vi "Main v0.1.vi"() -> ()   [LabVIEW 2017]
doc: "This template is for the Queued Message Handler design pattern.\n\nThe Event Handling Loop generates messages based on user interface actions.\n\nThe Message Handling Loop processes messages generated by the Event Handling Loop, or by other messages. The messages are string values, so new messages can be added easily to the Message Cases case structure in the Message Handling Loop. Each message cluster can also provide an optional value for Message Data, which is a variant that can be converted to whatever message-specific data is required."
uses:
  Controls/Main Tabs.ctl
  Controls/Auto.ctl
  Controls/UI Data.ctl
  support/Message Queue/Enqueue Message (Single).vi
  <vilib>/Utility/error.llb/Error Cluster From Error Code.vi
  <vilib>/ErrorRing/Error Ring.xnode
  support/Message Queue/Message Queue.lvlib
  support/User Event - Stop/User Event - Stop.lvlib
panel:
  out "Date-Time":string caption="Dip-Tube Assembly Automation (HMI) v0.1"
  out "Main Tab":T1
  in  "Autocycle":T2
  in  "Manual":bool
  in  "Parameters":bool
  in  "Maintenance":bool
  in  "Save Para":bool
  in  "Home Para":bool
  in  "ParaTab":T3(tab)
  in  "StopperRearDelay":dbl format="%#.2f"
  in  "StopperFrontDelay":dbl format="%#.2f"
  in  "MaxAlarms":dbl caption="Max Alarms in 1 Minute" format="%#.2f"
  in  "MaxConsecutive":dbl caption="Max Consecutive Alarms" format="%#.2f"
  in  "Gate Close Delay":dbl format="%#.2f"
  in  "Gate Open Delay":dbl format="%#.2f"
  in  "BF Off Delay":dbl format="%#.2f"
  in  "BF On Delay":dbl format="%#.2f"
  in  "DelayAfterReject":dbl format="%#.2f"
  in  "MeasurementTime":dbl format="%#.2f"
  in  "DelayAfterMesFront":dbl format="%#.2f"
  in  "DelayAfterCut":dbl format="%#.2f"
  in  "DelayAfterCutClamp":dbl format="%#.2f"
  in  "DelayAfterInsClamp":dbl format="%#.2f"
  in  "DelayToClose":dbl format="%#.2f"
  in  "DelayToOpen":dbl format="%#.2f"
  in  "DelayAfterInsertion":dbl format="%#.2f"
  in  "DelayBeforeInsertion":dbl format="%#.2f"
  in  "AgitatorUpTime":dbl format="%#.2f"
  in  "AgitatorDownTime":dbl format="%#.2f"
  in  "All IO":bool
  in  "Stats":bool
  in  "Home AC":bool
  out "Status":string
  out "Count":dbl format="%06.0f"
  out "Count 3":dbl caption="Cycle Time" format="%0.2f"
  out "Count 2":dbl caption="Rejects" format="%06.0f"
  in  "Statuses":string[][](table)
  in  "Exit":bool
  # "Vision Harmony Dip-Tube Assembly Automation"
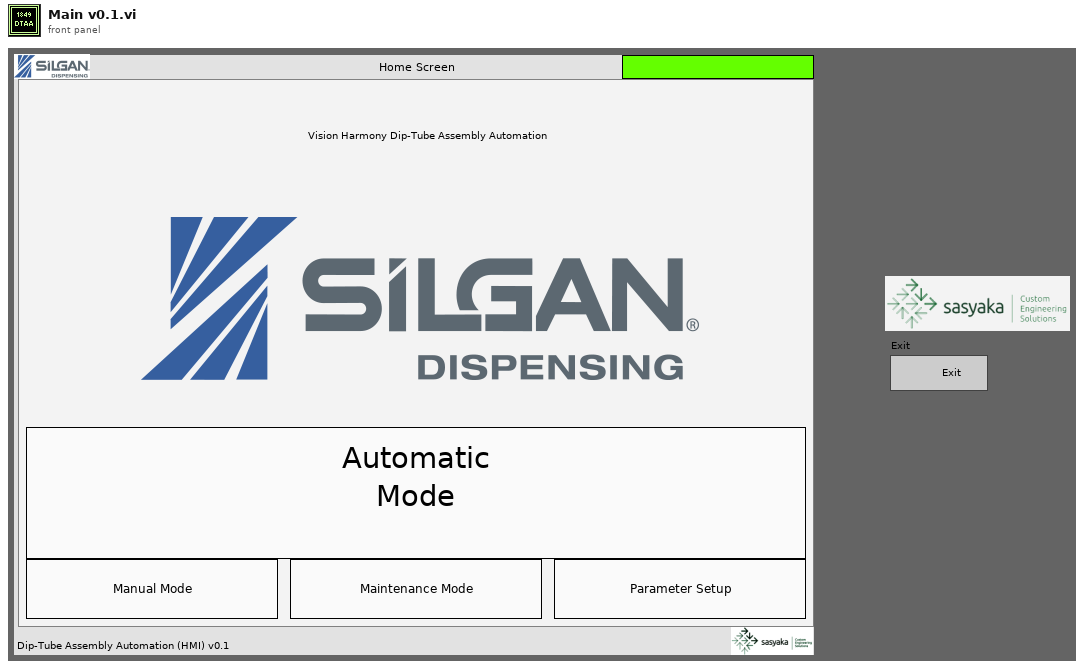
[diagram p1: front panel]
types:
  T1 = typedef "Main Tabs.ctl" = enum32{"Home Screen", "Parameter Setup", "Manual Mode", "Autocycle"}
  T2 = typedef "Auto.ctl" = bool
  T3 = enum32{"General & Indexing", "Bowl Feeder & Pump Conveyor", "Cutting, Measurement & Rejection", "Tube Feeder & Insertion"}
  T4 = typedef "UI Data.ctl" = cluster{"Main Tab":refnum<vi>}
  T5 = typedef "Message Queue.lvlib/All Message Queues.ctl" = cluster{"UI":refnum<queue>}
  T6 = enum8{"Enabled", "Disabled", "Disabled and Grayed Out"}
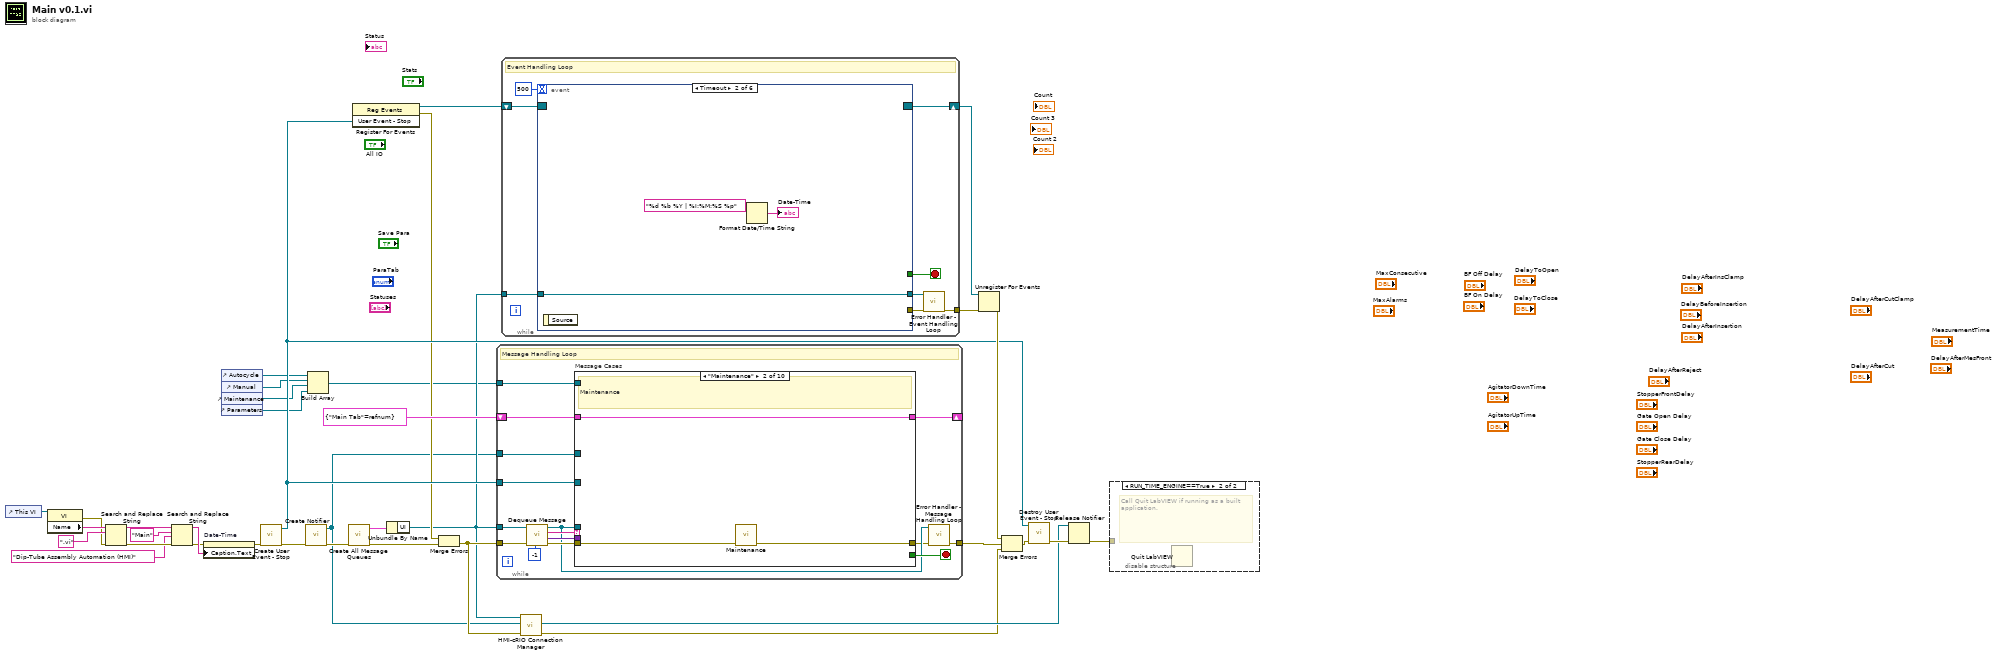
[diagram p0: block diagram]
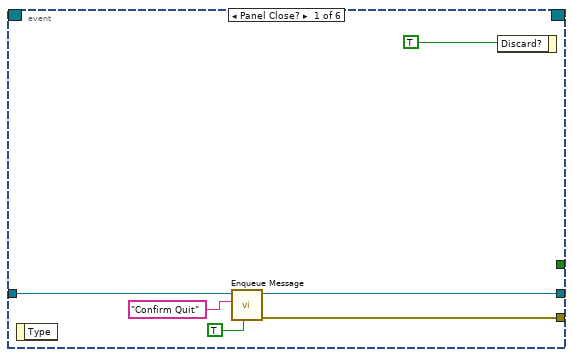
[diagram p2: hidden frame]
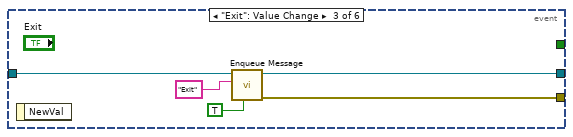
[diagram p3: hidden frame]
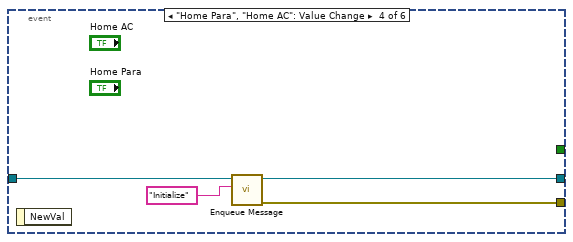
[diagram p4: hidden frame]
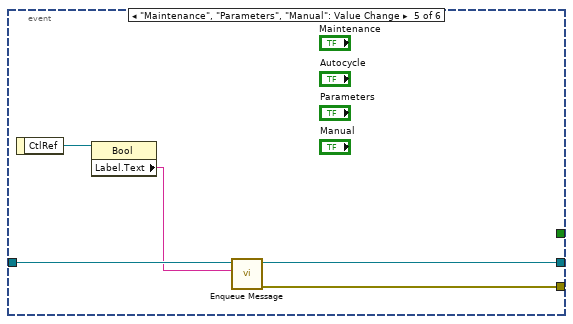
[diagram p5: hidden frame]
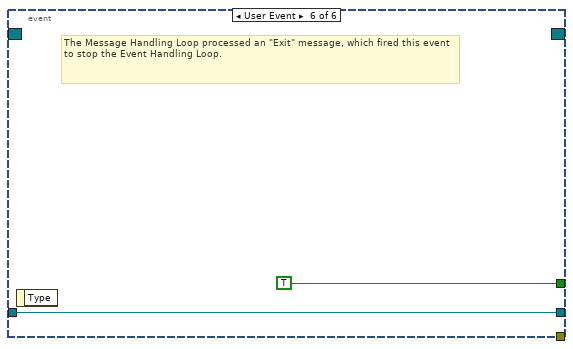
[diagram p6: hidden frame]
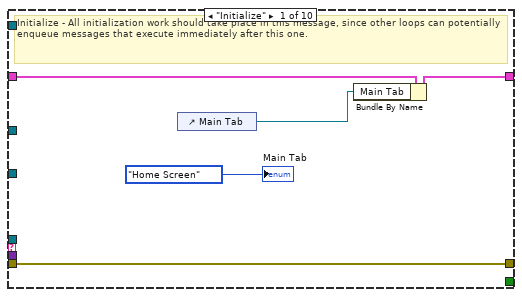
[diagram p7: hidden frame]
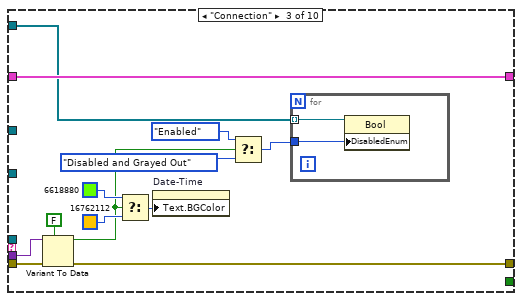
[diagram p8: hidden frame]
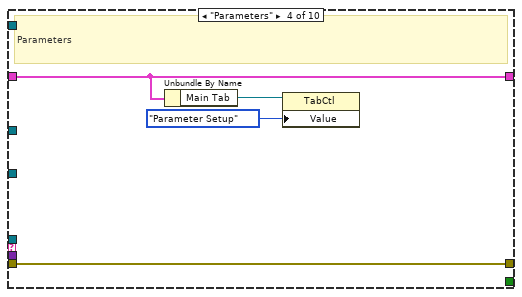
[diagram p9: hidden frame]
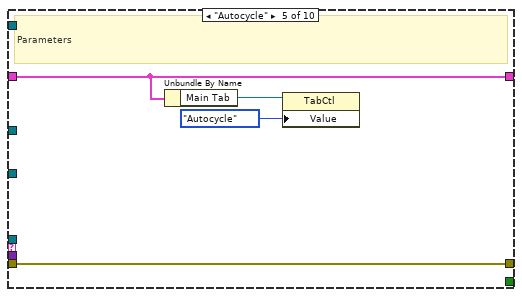
[diagram p10: hidden frame]
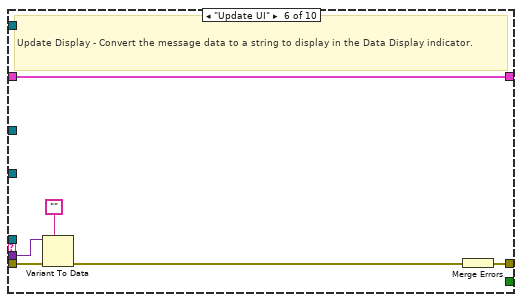
[diagram p11: hidden frame]
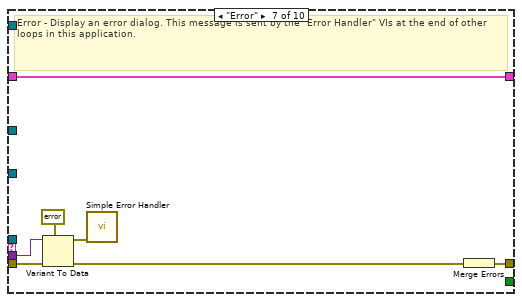
[diagram p12: hidden frame]
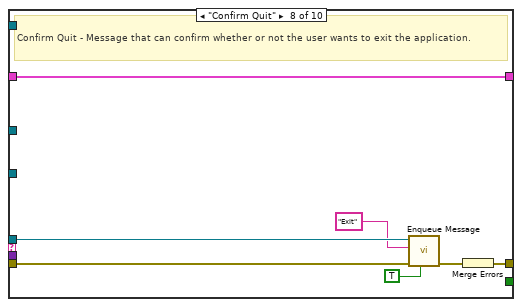
[diagram p13: hidden frame]
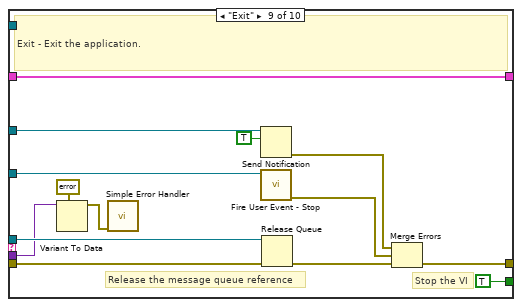
[diagram p14: hidden frame]
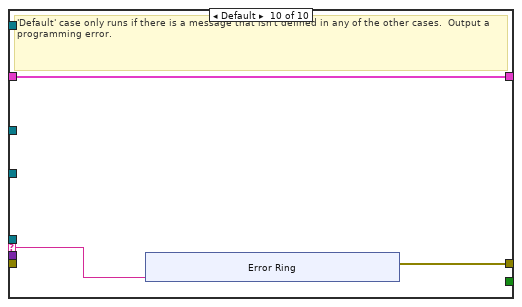
[diagram p15: hidden frame]
diagram:
  n1 = control-ref of="This VI"() -> (w5:refnum<vi>)
  n2 = property class="VI"(reference=w5) -> (error out=w4:errorcluster, "Name"=w11:string)  [unwired: 1 in, 1 out]
  n3 = Search and Replace String(input string=w11, search string=".vi", error in=w4) -> (result string=w9:string, error out=w8:errorcluster)  [unwired: 5 in, 2 out]
  n4 = Search and Replace String(input string=w9, search string="Main", replace string="Dip-Tube Assembly Automation (HMI)" ("replace string (\"\")"), error in=w8) -> (result string=w3:string, error out=w2:errorcluster)  [unwired: 4 in, 2 out]
  n5 = property on="Date-Time" class="Str"(error in=w2, "Caption.Text"=w3) -> (error out=w1:errorcluster)  [unwired: 1 in, 1 out]
  n6 = control-ref of="Autocycle"() -> (w16:refnum<vi>)
  n7 = control-ref of="Manual"() -> (w15:refnum<vi>)
  n8 = control-ref of="Maintenance"() -> (w14:refnum<vi>)
  n9 = control-ref of="Parameters"() -> (w13:refnum<vi>)
  n10 = call "Create User Event - Stop.vi"("error in (no error)"=w1) -> ("error out"=w23:errorcluster, "User Event - Stop"=w27:refnum<user-event>)  [unwired: 9 in]
  n11 = call "Create Notifier.vi"("error in (no error)"=w23) -> ("error out"=w22:errorcluster, "notifier out"=w17:refnum<notifier>)  [unwired: 9 in]
  n12 = Build Array(w16, w15, w14, w13) -> (w12:refnum<vi>[])
  n13 = call "Create All Message Queues.vi"("error in (no error)"=w22) -> ("error out"=w36:errorcluster, "Message Queues out"=w35:T5)  [unwired: 9 in]
  n14 = register-events(w27) -> (reference out=w28:refnum<event-registration>, error out=w26:errorcluster)  [unwired: 2 in]
  n15 = Unbundle By Name(w35) -> ("UI"=w24:refnum<queue>)
  n16 = Merge Errors(w26, w36) -> (w25:errorcluster)
  n17 = while {
    tunnel: w24 -> [w43]
    shift-right: [w50] -> _
    shift-left: T4 {"Main Tab"=refnum} ("Data Cluster") -> [w51]
    tunnel: w27 -> [w48]
    tunnel: w25 -> [w47]
    tunnel: [w41] -> w34
    tunnel: w17 -> [w38]
    tunnel: w12 -> [w37]
    stop <- w49 stop-if-true
    # "Message Handling Loop"
    n18 = call "Dequeue Message.vi"("timeout"=-1, "error in (no error)"=w47, "Message Queue"=w43) -> ("error out"=w46:errorcluster, "Message Data"=w44:variant, "Message"=w45:string, "dup Message Queue"=w42:refnum<queue>)  [unwired: 5 in]
    n19 = case "Message Cases" shown="\"Maintenance\"" w45 {
      selector: w45 -> [_ _ _ _ _ _ _ _ _ w117]
      tunnel: w42 -> [_ _ _ _ _ _ _ w98 w116 _]
      tunnel: w46 -> [w56 w58 w70 w78 w82 w86 w95 w102 w109 _]
      tunnel: [w56 w57 w69 w78 w82 w87 w89 w100 w112 w118] -> w40
      tunnel: w51 -> [w55 w59 w72 w77 w81 w88 w94 w101 w115 w119]
      tunnel: [w54 w59 w72 w77 w81 w88 w94 w101 w115 w119] -> w50
      tunnel: [_ _ _ _ _ _ _ _ TRUE _] -> w49
      tunnel: w44 -> [_ _ w68 _ _ w85 w93 _ w106 _]
      tunnel: w48 -> [_ _ _ _ _ _ _ _ w111 _]
      tunnel: w38 -> [_ _ _ _ _ _ _ _ w105 _]
      tunnel: w37 -> [_ _ w64 _ _ _ _ _ _ _]
      frame "Initialize" {
        # "Initialize - All initialization work should take place in this message, since other loops can potentially enqueue messages that execute immediately after this one."
        n20 = control-ref of="Main Tab"() -> (w53:refnum<vi>)
        n21 = Bundle By Name(cluster=w55, "Main Tab"=w53) -> (w54:T4)
        "Main Tab" <- Main_Tabs."Home Screen" ("Main Tab")
      }
      frame "Maintenance" {
        # "Maintenance"
        n22 = call "Maintenance.vi"("Error In"=w58) -> ("Error out"=w57:errorcluster)  [unwired: 10 in]
      }
      frame "Connection" {
        n23 = Variant To Data(error in=w70, type=FALSE, Variant=w68) -> (data=w63:bool, error out=w69:errorcluster)
        n24 = Select(t=u32 6618880 ("Text.Text Colors:BG Color"), s=w63, f=u32 16762112 ("Text.Text Colors:BG Color")) -> (s? t:f=w65:u32)
        n25 = property on="Date-Time" class="Str"("Text.BGColor"=w65) -> ()  [unwired: 2 in, 2 out]
        n26 = Select(t=T6."Enabled" ("Disabled"), s=w63, f=T6."Disabled and Grayed Out") -> (s? t:f=w61:T6)
        n27 = for {
          tunnel: w64 -> [w74] mode=indexing
          tunnel: w61 -> [w73]
          n28 = property class="Bool"(reference=w74, "DisabledEnum"=w73) -> ()  [unwired: 1 in, 2 out]
        }
      }
      frame "Parameters" {
        # "Parameters"
        n29 = Unbundle By Name(w77) -> ("Main Tab"=w76:refnum<vi>)
        n30 = property class="TabCtl"(reference=w76, "Value"=Main_Tabs."Parameter Setup" ("Main Tab")) -> ()  [unwired: 1 in, 2 out]
      }
      frame "Autocycle" {
        # "Parameters"
        n31 = Unbundle By Name(w81) -> ("Main Tab"=w80:refnum<vi>)
        n32 = property class="TabCtl"(reference=w80, "Value"=Main_Tabs."Autocycle" ("Main Tab")) -> ()  [unwired: 1 in, 2 out]
      }
      frame "Update UI" {
        # "Update Display - Convert the message data to a string to display in the Data Display indicator."
        n33 = Variant To Data(error in=w86, type="", Variant=w85) -> (error out=w83:errorcluster)  [unwired: 1 out]
        n34 = Merge Errors(w83) -> (w87:errorcluster)
      }
      frame "Error" {
        # "Error - Display an error dialog. This message is sent by the \"Error Handler\" VIs at the end of other loops in this application."
        n35 = Variant To Data(error in=w95, type=errorcluster {"status"=FALSE, "code"=0, "source"=""} ("error constant"), Variant=w93) -> (data=w91:errorcluster, error out=w90:errorcluster)
        n36 = call <vilib>:"Simple Error Handler.vi"("error in (no error)"=w91) -> ()  [unwired: 4 in, 5 out]
        n37 = Merge Errors(w90) -> (w89:errorcluster)
      }
      frame "Confirm Quit" {
        # "Confirm Quit - Message that can confirm whether or not the user wants to exit the application."
        n38 = call-poly "Enqueue Message.vi"("Priority Message? (F)"=TRUE, "error in (no error)"=w102, "Message"="Exit", "Message Queue"=w98) -> ("error out"=w99:errorcluster)  [unwired: 6 in, 1 out]
        n39 = Merge Errors(w99) -> (w100:errorcluster)
      }
      frame "Exit" {
        # "Stop the VI"
        # "Release the message queue reference"
        # "Exit - Exit the application."
        n40 = Variant To Data(type=errorcluster {"status"=FALSE, "code"=0, "source"=""} ("error constant"), Variant=w106) -> (data=w107:errorcluster)  [unwired: 1 in, 1 out]
        n41 = call <vilib>:"Simple Error Handler.vi"("error in (no error)"=w107) -> ()  [unwired: 4 in, 5 out]
        n42 = Send Notification(notification=TRUE, notifier=w105) -> (error out=w103:errorcluster)  [unwired: 1 in, 1 out]
        n43 = call "Fire User Event - Stop.vi"("User Event - Stop"=w111) -> ("error out"=w110:errorcluster)  [unwired: 10 in]
        n44 = Release Queue(queue=w116, error in (no error)=w109) -> (error out=w113:errorcluster)  [unwired: 1 in, 2 out]
        n45 = Merge Errors(w103, w110, w113) -> (w112:errorcluster)
      }
      frame Default {
        # "'Default' case only runs if there is a message that isn't defined in any of the other cases.  Output a programming error."
        n46 = xnode "Error Ring"("parameter 0"=w117) -> ("error out"=w118:errorcluster)
      }
    }
    n47 = call "Error Handler - Message Handling Loop.vi"("error in (no error)"=w40, "Message Queue"=w42) -> ("dup error in"=w41:errorcluster)  [unwired: 8 in, 1 out]
  }
  n48 = while {
    tunnel: w24 -> [w134]
    shift-right: [w132] -> w31
    shift-left: w28 -> [w133]
    tunnel: [w128] -> w29
    stop <- w130 stop-if-true
    # "Event Handling Loop"
    n49 = event shown="[1] Timeout" {
      selector: w133 -> [_ _ _ _ _ _]
      dyn-events: [_ _ _ _ _ _] -> w132
      timeout: 500 -> [_ _ _ _ _ _]
      tunnel: [_ _ _ _ _ TRUE ("Discard?")] -> w130
      tunnel: w134 -> [w139 w143 w148 w152 w157 w159]
      tunnel: [w138 _ w147 w151 w156 _] -> w131
      tunnel: [w137 w143 w146 w150 w155 w159] -> w129
      event Panel Close? {
        n50 = event-data() -> ()  [unwired: 1 in, 1 out]
        n51 = call-poly "Enqueue Message.vi"("Priority Message? (F)"=TRUE, "Message"="Confirm Quit", "Message Queue"=w139) -> ("error out"=w138:errorcluster, "dup Message Queue"=w137:refnum<queue>)  [unwired: 7 in]
        n52 = event-data("Discard?"=TRUE) -> ()  [unwired: 1 in, 1 out]
      }
      event Timeout {
        n53 = event-data() -> ()  [unwired: 1 in, 1 out]
        n54 = Format Date/Time String(time format string (%c)="%d %b %Y | %I:%M:%S %p") -> (date/time string=→"Date-Time":string)  [unwired: 2 in]
      }
      event "Exit": Value Change {
        n55 = event-data() -> ()  [unwired: 1 in, 1 out]
        n56 = call-poly "Enqueue Message.vi"("Priority Message? (F)"=TRUE, "Message"="Exit", "Message Queue"=w148) -> ("error out"=w147:errorcluster, "dup Message Queue"=w146:refnum<queue>)  [unwired: 7 in]
      }
      event "Home Para", "Home AC": Value Change {
        n57 = event-data() -> ()  [unwired: 1 in, 1 out]
        n58 = call-poly "Enqueue Message.vi"("Message"="Initialize", "Message Queue"=w152) -> ("error out"=w151:errorcluster, "dup Message Queue"=w150:refnum<queue>)  [unwired: 8 in]
      }
      event "Maintenance", "Parameters", "Manual": Value Change {
        n59 = event-data() -> ("CtlRef"=w154:refnum<vi>)  [unwired: 1 in]
        n60 = property class="Bool"(reference=w154) -> ("Label.Text"=w153:string)  [unwired: 1 in, 2 out]
        n61 = call-poly "Enqueue Message.vi"("Message"=w153, "Message Queue"=w157) -> ("error out"=w156:errorcluster, "dup Message Queue"=w155:refnum<queue>)  [unwired: 8 in]
      }
      event User Event {
        # "The Message Handling Loop processed an \"Exit\" message, which fired this event to stop the Event Handling Loop."
        n62 = event-data() -> ()  [unwired: 1 in, 1 out]
      }
    }
    n63 = call "Error Handler - Event Handling Loop.vi"("error in (no error)"=w131, "Message Queue"=w129) -> ("dup error in"=w128:errorcluster)  [unwired: 8 in, 1 out]
  }
  n64 = call "HMI-cRIO Connection Manager.vi"("error in"=w25, "notifier in"=w17, "Queue in"=w24) -> ("error out"=w18:errorcluster, "Notifier out"=w19:refnum<notifier>)  [unwired: 7 in]
  n65 = Unregister For Events(event registration refnum=w31, error in=w29) -> (error out=w32:errorcluster)
  n66 = Merge Errors(w32, w34, w18) -> (w33:errorcluster)
  n67 = call "Destroy User Event - Stop.vi"("error in (no error)"=w33, "User Event - Stop"=w27) -> ("error out"=w21:errorcluster)  [unwired: 9 in]
  n68 = Release Notifier(notifier=w19, error in (no error)=w21) -> (error out=w20:errorcluster)  [unwired: 1 in, 2 out]
  n69 = disable-structure shown="RUN_TIME_ENGINE==True" {
    disable-tunnel: w20 -> [_ _]
    frame condition #0 (active) {
    }
    frame condition #1 {
      # "Call Quit LabVIEW if running as a built application."
      n70 = Quit LabVIEW() -> ()  [unwired: 1 in]
    }
  }
